vi "power spectrum fourier.vi"(7 "PSD (T) PS (F)":bool, 9 "starting frequency bin to plot":i32, 10 "Array":sgl[](array[numeric]), 11 "rep rate (Hz)":sgl) -> (3 "Power Spectrum":cluster{"f0":dbl, "df":dbl, "magnitude":dbl[]})   [LabVIEW 2020]
uses:
  <vilib>/Analysis/baseanly.llb/Mean (DBL).vi
  <vilib>/express/express analysis/Spectral/Block/exnSpectralBlock spectral measurements PSD poly.vi
  <vilib>/express/express analysis/Spectral/Block/exnSpectralBlock spectral measurements PSD WFM.vi
  <vilib>/express/express analysis/Spectral/Block/exnSpectralBlock spectral measurements power poly.vi
  <vilib>/express/express analysis/Spectral/Block/exnSpectralBlock spectral measurements power WFM.vi
  <vilib>/express/express analysis/Spectral/XNode/ExpressSpectralMeasurementsBlockNode.xnode
  <vilib>/Analysis/NI_AALPro.lvlib
  <vilib>/Analysis/2dsp.llb/Power Spectrum (DBL).vi
  <vilib>/measure/NI_MAPro.lvlib
  <vilib>/Analysis/NI_AALBase.lvlib
panel:
  out "df":sgl
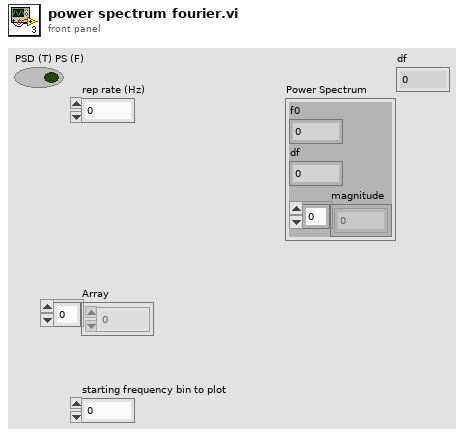
[diagram p1: front panel]
types:
  T1 = cluster{"averaging mode":u16, "weighting mode":u16, "number of averages":u32}
  T2 = cluster{"dB On (F)":bool, "unwrap phase (F)":bool, "convert to degree (F)":bool}
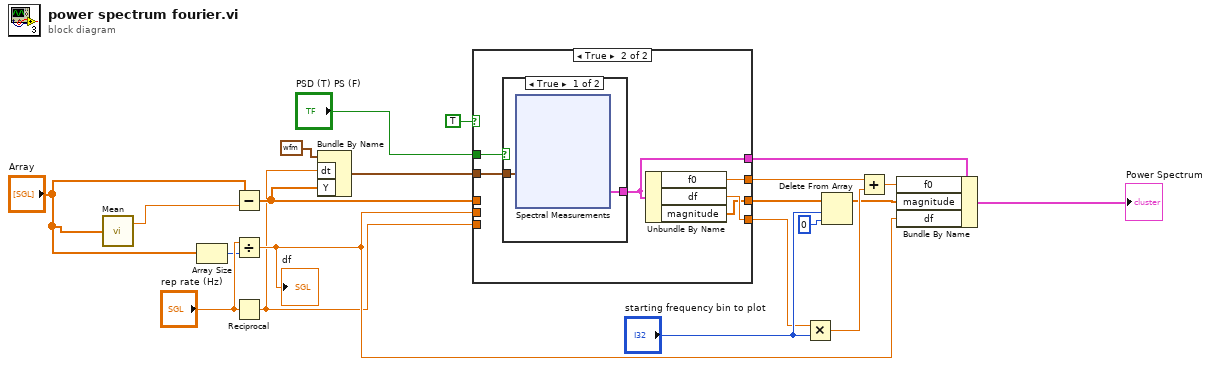
[diagram p0: block diagram]
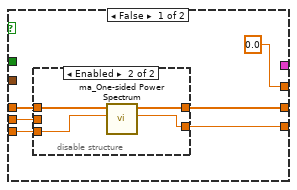
[diagram p2: hidden frame]
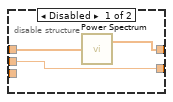
[diagram p3: hidden frame]
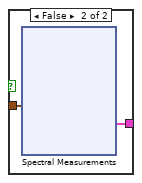
[diagram p4: hidden frame]
diagram:
  n1 = call-poly <vilib>:"Mean.vi"("X"="Array") -> ("mean"=w2:dbl)  [unwired: 1 out]
  n2 = Array Size(array="Array") -> (size(s)=w8:i32)
  n3 = Subtract(x="Array", y=w2) -> (x-y=w6:dbl[])
  n4 = Divide(x="rep rate (Hz)", y=w8) -> (x/y=w5:sgl)
  "df" <- w5
  n5 = Reciprocal(x="rep rate (Hz)") -> (1/x=w4:sgl)
  n6 = Bundle By Name(cluster=waveform(dbl) {"t0"=timestamp(0 s since 1904-01-01), "dt"=0.0, "Y"=[]} ("Signals"), "dt"=w4, "Y"=w6) -> (w10:waveform(dbl))
  n7 = case shown="True" TRUE {
    tunnel: [w23 w40] -> w19
    tunnel: [_ w39] -> w15
    tunnel: [w26 w38] -> w13
    tunnel: [0.0 ("f0") w37] -> w12
    tunnel: w10 -> [_ w36]
    tunnel: w6 -> [w27 _]
    tunnel: w5 -> [w22 _]
    tunnel: w4 -> [w24 _]
    tunnel: "PSD (T) PS (F)" -> [_ w35]
    frame False {
      n8 = disable-structure shown="Enabled" {
        disable-tunnel: w27 -> [w30 w34]
        disable-tunnel: [w29 w32] -> w26
        disable-tunnel: w24 -> [_ w33]
        disable-tunnel: [w28 w31] -> w23
        disable-tunnel: w22 -> [w28 _]
        frame Disabled {
          n9 = call-poly <vilib>:"Power Spectrum.vi"("X"=w30) -> ("Power Spectrum"=w29:dbl[])  [unwired: 1 out]
        }
        frame Enabled {
          n10 = call <vilib>:"ma_One-sided Power Spectrum.vi"("dt"=w33, "signal (V)"=w34) -> ("df"=w31:dbl, "power spectrum (V^2 rms)"=w32:dbl[])  [unwired: 1 in, 7 out]
        }
      }
    }
    frame True {
      n11 = case shown="True" w35 {
        tunnel: [w42 w53] -> w39
        tunnel: w36 -> [w41 w52]
        frame True {
          n12 = xnode "Spectral Measurements"("Signals"=w41) -> ("PSD"=w42:cluster{"f0":dbl, "df":dbl, "magnitude":dbl[]})  [unwired: 1 in, 1 out]
        }
        frame False {
          n13 = xnode "Spectral Measurements"("Signals"=w52) -> ("Power Spectrum"=w53:cluster{"f0":dbl, "df":dbl, "magnitude":dbl[]})  [unwired: 1 in, 1 out]
        }
      }
      n14 = Unbundle By Name(w39) -> ("f0"=w37:dbl, "df"=w40:dbl, "magnitude"=w38:dbl[])
    }
  }
  n15 = Multiply(x=w19, y="starting frequency bin to plot") -> (x*y=w20:dbl)
  n16 = Delete From Array(array=w13, length="starting frequency bin to plot", index=0) -> (array with subset deleted=w17:dbl[])  [unwired: 1 out]
  n17 = Add(x=w12, y=w20) -> (x+y=w16:dbl)
  n18 = Bundle By Name(cluster=w15, "f0"=w16, "magnitude"=w17, "df"=w5) -> (→"Power Spectrum":cluster{"f0":dbl, "df":dbl, "magnitude":dbl[]})
